vi "Run.vi"(8 "error in (no error)":errorcluster caption="entrée d'erreur (pas d'erreur)", 9 "X":string[][](array[string]), 10 "Type X":T2(ring), 11 "binarize.lvclass":refnum<class "binarize.lvclass">) -> (0 "error out":errorcluster caption="sortie d'erreur", 2 "Data":T1, 3 "binarize.lvclass":refnum<class "binarize.lvclass">)   [LabVIEW 2020, in "binarize.lvclass"]
uses:
  binarize.lvclass
  binarize.lvclass/binarize.ctl
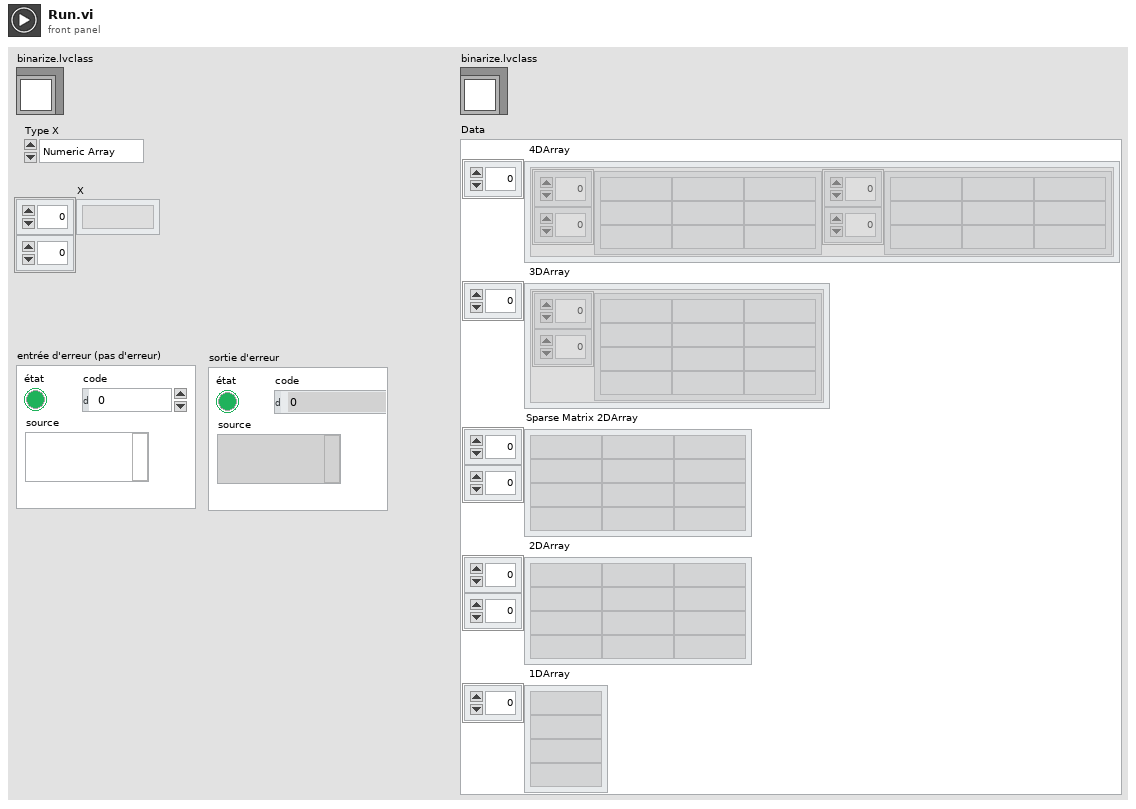
[diagram p1: front panel]
types:
  T1 = cluster{" 4DArray":cluster{"1":string[][], "2":string[][]}[], " 3DArray":cluster{"Tableau":string[][]}[], "Sparse Matrix 2DArray":string[][], " 2DArray":string[][], " 1DArray":string[]}
  T2 = enum16{"Numeric Array", "String Array", "Sparse"}
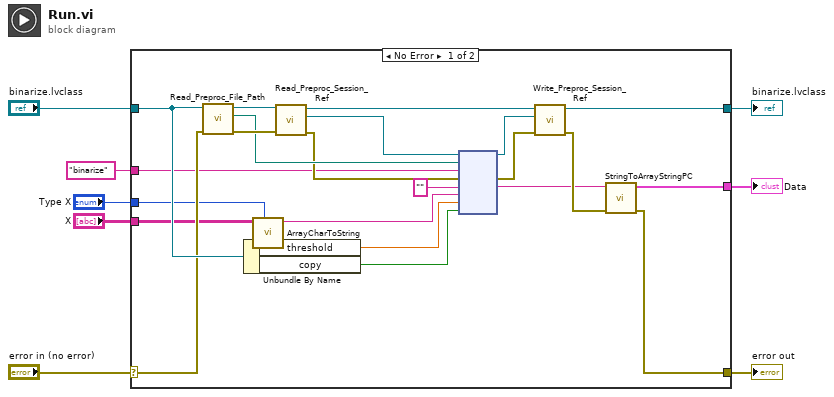
[diagram p0: block diagram]
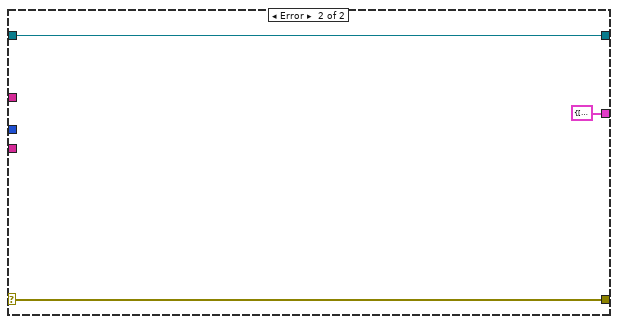
[diagram p2: hidden frame]
diagram:
  n1 = case shown="No Error" "error in (no error)" {
    selector: "error in (no error)" -> [w18 w33]
    tunnel: [w10 w33] -> w7
    tunnel: [w9 w32] -> w5
    tunnel: "binarize.lvclass" -> [w19 w32]
    tunnel: "binarize" ("Fonction") -> [w17 _]
    tunnel: [w11 T1 {" 4DArray"=[], " 3DArray"=[], "Sparse Matrix 2DArray"=[], " 2DArray"=[], " 1DArray"=[]} ("Data")] -> w1
    tunnel: "X" -> [w15 _]
    tunnel: "Type X" -> [w16 _]
    frame No Error {
      n2 = call-dynamic "Read_Preproc_File_Path.vi"("error in (no error)"=w18, "Python in"=w19) -> ("error out"=w29:errorcluster, "File_Path"=w26:path, "Python out"=w30:refnum<class "binarize.lvclass">)  [unwired: 7 in]
      n3 = Unbundle By Name(w19) -> ("threshold"=w21:dbl, "copy"=w20:bool)
      n4 = call "ArrayCharToString.vi"("Type"=w16, "TAB"=w15) -> ("Instruction"=w14:string)  [unwired: 9 in]
      n5 = call-dynamic "Read_Preproc_Session_Ref.vi"("error in (no error)"=w29, "Python in"=w30) -> ("error out"=w25:errorcluster, "Session_ref"=w27:refnum<k35>, "Python out"=w28:refnum<class "binarize.lvclass">)  [unwired: 7 in]
      n6 = node(w27, w26, w17, w25, "", w14, w21, w20) -> (w23:refnum<k35>, w24:errorcluster, w12:string)  [unwired: 3 in, 2 out]
      n7 = call-dynamic "Write_Preproc_Session_Ref.vi"("error in (no error)"=w24, "Session_ref"=w23, "Python in"=w28) -> ("error out"=w13:errorcluster, "Python out"=w9:refnum<class "binarize.lvclass">)  [unwired: 7 in]
      n8 = call "StringToArrayStringPC.vi"("sortie d'erreur"=w13, "Return value"=w12) -> ("sortie d'erreur"=w10:errorcluster, "Data"=w11:T1)  [unwired: 8 in]
    }
    frame Error {
    }
  }
  "error out" <- w7
  "binarize.lvclass" <- w5
  "Data" <- w1
